vi "Write nextInChain.vi"(8 "error in (no error)":errorcluster, 10 "Chain.lvclass":refnum<class "Chain.lvclass">, 11 "Divide in":refnum<class "Divide.lvclass">) -> (0 "error out":errorcluster, 3 "Divide out":refnum<class "Divide.lvclass">)   [LabVIEW 2018, in "Divide.lvclass"]
uses:
  Divide.lvclass
  Chain Class/Chain.lvclass
  Divide.lvclass/Divide.ctl
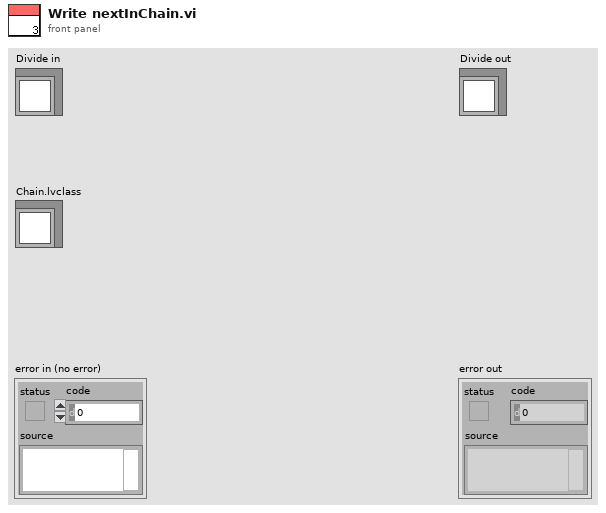
[diagram p1: front panel]
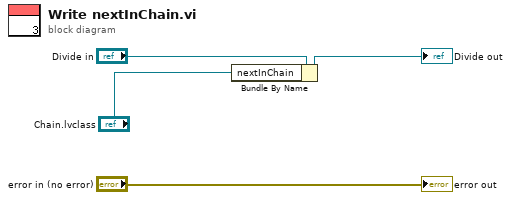
[diagram p0: block diagram]
diagram:
  n1 = Bundle By Name(cluster="Divide in", "nextInChain"="Chain.lvclass") -> (→"Divide out":refnum<class "Divide.lvclass">)
  "error out" <- "error in (no error)"
